vi "Read INI File.vi"(8 "error in":errorcluster, 11 "INI File":path) -> (0 "error out":errorcluster, 2 "File paths":T1, 3 "INI refnum":T2)   [LabVIEW 2025, in "Config Tool.lvlib"]
uses:
  Config Tool.lvlib
  <vilib>/Utility/config.llb/Config Data RefNum.ctl
  Controls/FilePaths.ctl
  <vilib>/Utility/config.llb/Read Key (Path).vi
  <vilib>/Utility/config.llb/NI_LVConfig.lvlib
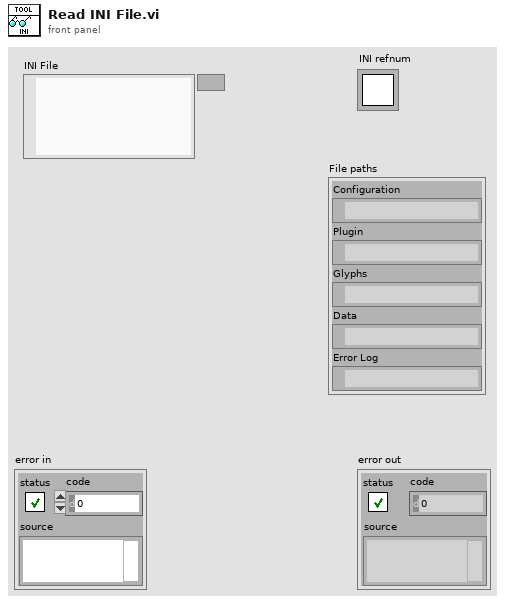
[diagram p1: front panel]
types:
  T1 = typedef "Config Tool.lvlib/FilePaths.ctl" = cluster{"Configuration":path, "Plugin":path, "Glyphs":path, "Data":path, "Error Log":path}
  T2 = typedef "NI_LVConfig.lvlib/Config Data RefNum.ctl" = refnum<k1>
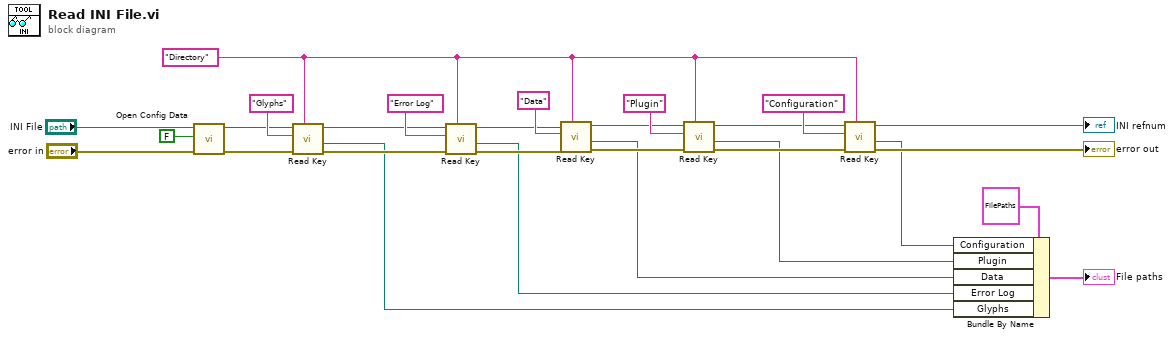
[diagram p0: block diagram]
diagram:
  w3 = "Directory" ("section")
  n1 = call <vilib>:"Open Config Data.vi"("error in (no error)"="error in", "create file if necessary (T)"=FALSE, "configuration file path"="INI File") -> ("error out"=w4:errorcluster, "refnum"=w5:T2)  [unwired: 6 in, 1 out]
  n2 = call-poly <vilib>:"Read Key.vi"("section"=w3, "error in (no error)"=w4, "key"="Glyphs", "refnum"=w5) -> ("error out"=w13:errorcluster, "value"=w6:path, "refnum out"=w14:T2)  [unwired: 4 in, 1 out]
  n3 = call-poly <vilib>:"Read Key.vi"("section"=w3, "error in (no error)"=w13, "key"="Error Log", "refnum"=w14) -> ("error out"=w12:errorcluster, "value"=w7:path, "refnum out"=w11:T2)  [unwired: 4 in, 1 out]
  n4 = call-poly <vilib>:"Read Key.vi"("section"=w3, "error in (no error)"=w12, "key"="Data", "refnum"=w11) -> ("error out"=w19:errorcluster, "value"=w8:path, "refnum out"=w20:T2)  [unwired: 4 in, 1 out]
  n5 = call-poly <vilib>:"Read Key.vi"("section"=w3, "error in (no error)"=w19, "key"="Plugin", "refnum"=w20) -> ("error out"=w25:errorcluster, "value"=w9:path, "refnum out"=w24:T2)  [unwired: 4 in, 1 out]
  n6 = call-poly <vilib>:"Read Key.vi"("section"=w3, "error in (no error)"=w25, "key"="Configuration", "refnum"=w24) -> ("error out"=→"error out":errorcluster, "value"=w10:path, "refnum out"=→"INI refnum":T2)  [unwired: 4 in, 1 out]
  n7 = Bundle By Name(cluster=T1 {"Configuration"=path "", "Plugin"=path "", "Glyphs"=path "", "Data"=path "", "Error Log"=path ""} ("File paths"), "Configuration"=w10, "Plugin"=w9, "Data"=w8, "Error Log"=w7, "Glyphs"=w6) -> (→"File paths":T1)
